vi "InsertBadDependency.vi"(8 "error in (no error)":errorcluster, 9 "Dependency items":refnum<class "ILabVIEWItem.lvclass">[](array[class]), 10 "ILabVIEWItem":refnum<class "ILabVIEWItem.lvclass">, 11 "CReporter in":refnum<class "CReporter.lvclass">) -> (0 "error out":errorcluster, 3 "CReporter out":refnum<class "CReporter.lvclass">)   [LabVIEW 2020, in "DependencyInspection.lvlib" / "CReporter.lvclass"]
uses:
  CReporter.lvclass
  obj/Addons/LabVIEWObjectInterfaces.lvlibp/LabVIEWObjectInterfaces/ILabVIEWItem/ILabVIEWItem.lvclass
  CReporter.lvclass/CReporter.ctl
  CDependencyList/CDependencyList.lvclass
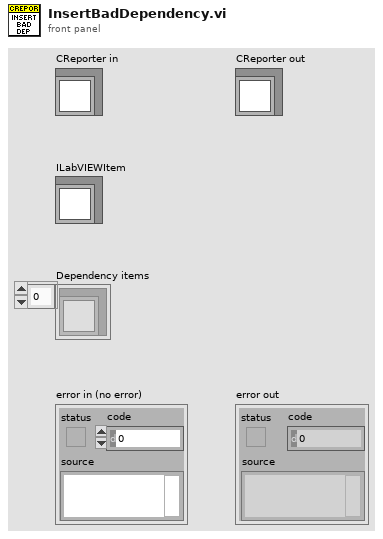
[diagram p1: front panel]
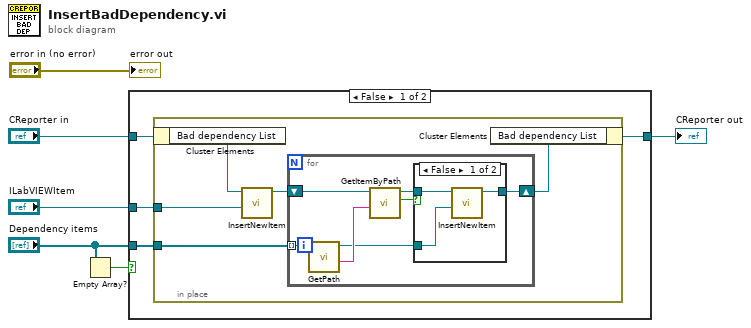
[diagram p0: block diagram]
diagram:
  n1 = Empty Array?(array="Dependency items") -> (empty?=w2:bool)
  n2 = case shown="False" w2 {
    tunnel: "CReporter in" -> [w10 w27]
    tunnel: [w9 w27] -> w4
    tunnel: "ILabVIEWItem" -> [w8 _]
    tunnel: "Dependency items" -> [w7 _]
    frame False {
      n3 = in-place {
        in-place-border: w8 -> [w14]
        in-place-border: w7 -> [w11]
        n4 = in-place-cluster #1(w10) -> ("Bad dependency List"=w15:refnum<class "CDependencyList.lvclass">)
        n5 = call-dynamic "InsertNewItem.vi"("ILabVIEWItem in"=w14, "CDependencyList in"=w15) -> ("CDependencyList out"=w13:refnum<class "CDependencyList.lvclass">)  [unwired: 7 in, 2 out]
        n6 = for {
          shift-right: [w19] -> w12
          shift-left: w13 -> [w22]
          tunnel: w11 -> [w21] mode=indexing
          n7 = call-dynamic "GetPath.vi"("ILabVIEWItem in"=w21) -> ("Path"=w20:string, "ILabVIEWItem out"=w16:refnum<class "ILabVIEWItem.lvclass">)  [unwired: 8 in, 1 out]
          n8 = call-dynamic "GetItemByPath.vi"("Path"=w20, "CDependencyList in"=w22) -> ("key found?"=w17:bool, "CDependencyList out"=w18:refnum<class "CDependencyList.lvclass">)  [unwired: 6 in, 2 out]
          n9 = case shown="False" w17 {
            tunnel: [w24 w26] -> w19
            tunnel: w18 -> [w25 w26]
            tunnel: w16 -> [w23 _]
            frame False {
              n10 = call-dynamic "InsertNewItem.vi"("ILabVIEWItem in"=w23, "CDependencyList in"=w25) -> ("CDependencyList out"=w24:refnum<class "CDependencyList.lvclass">)  [unwired: 7 in, 2 out]
            }
            frame True {
            }
          }
        }
        n11 = in-place-cluster #1("Bad dependency List"=w12) -> (w9:refnum<class "CReporter.lvclass">)
      }
    }
    frame True {
    }
  }
  "CReporter out" <- w4
  "error out" <- "error in (no error)"
